vi "LuaVIEW Register and Set Indexed Function.vi"(5 "LuaVIEW reference in":T1, 7 "index":i32, 9 "synopsis":string, 11 "error in (no error)":errorcluster) -> (6 "LuaVIEW reference out":T1, 15 "error out":errorcluster)   [LabVIEW 2012]
doc: "Registers an indexed function with the LuaVIEW state's private function registry and sets the function as part of the state's variable space so that it can be called by name. Indexed functions are functions whose LabVIEW-side functionality is specified via an index instead of a function VI reference. When an indexed function is called, \"LuaVIEW Execute Iteration\" will return and leave the handling to its caller. Thus, indexed functions can be implemented as part of anything that allows selection via an index (typically a case of a case structure)."
uses:
  typedefs/t_LuaVIEW Reference.ctl
  typedefs/et_LuaVIEW CIN Actions.ctl
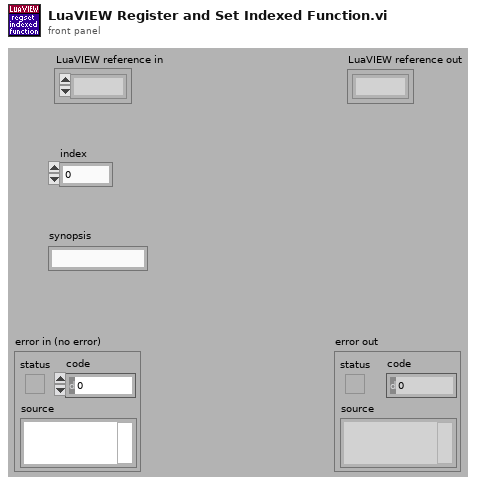
[diagram p1: front panel]
types:
  T1 = typedef "t_LuaVIEW Reference.ctl" = refnum<k1>
  T2 = typedef "et_LuaVIEW CIN Actions.ctl" = enum16{"checksynopsis", "_open", "_registerpublic", "_registerexport", "__never_an_error_result_ns", "luaversion", "cinversion", "_totals", "_taskcount", "pathological", "_unregnextpublic", "registryusecount", "__per_state_actions", "regsetprivate", "regsetindex", "regsetmodule", "_revokeexports", "_usepublic", "prepare", "compile", "execute", "call", "unregstaterefs", "_close", "pullboolean", "pullnumber", "pullI8", "pullU8", "pullI16", "pullU16", "pullI32", "pullU32", "pullobject", "pullrefnum", "pullstring", "pullflat", "pushflat", "pushobject", "getattribute", "setattribute", "stacktostring", "_startyieldtest", "_endyieldtest", "_pollprintbuffer", "__never_an_error_result_ps", "_pollexport", "setclone", "forcecleanup", "gettop", "clearstack", "insert", "pushboolean", "pushnumber", "pushrefnum", "pushstring", "pushnil", "pushvalue", "gettaskref", "settaskref"}
  T3 = typedef "et_LuaVIEW CIN Results.ctl" = enum16{"OK", "error", "main", "call", "clonecall", "modulecall", "exportcall", "index", "yield"}
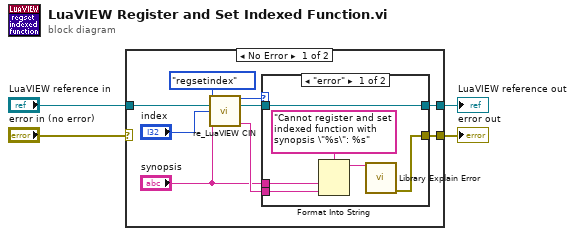
[diagram p0: block diagram]
diagram:
  n1 = case shown="No Error" "error in (no error)" {
    selector: "error in (no error)" -> [_ w22]
    tunnel: [w9 w21] -> w4
    tunnel: [w5 w22] -> w3
    tunnel: "LuaVIEW reference in" -> [w8 w21]
    frame No Error {
      n2 = call "re_LuaVIEW CIN.vi"("action"=et_LuaVIEW_CIN_Actions."regsetindex", "LuaVIEW reference in"=w8, "index in"="index", "string in"="synopsis") -> ("result"=w12:T3, "LuaVIEW reference out"=w10:T1, "string out"=w11:string)  [unwired: 5 in, 4 out]
      n3 = case shown="\"error\"" w12 {
        tunnel: w11 -> [w18 _]
        tunnel: [w19 _] -> w5
        tunnel: "synopsis" -> [w17 _]
        tunnel: w10 -> [w14 w20]
        tunnel: [w14 w20] -> w9
        frame "error" {
          n4 = Format Into String(format string="Cannot register and set indexed function with  synopsis \"%s\": %s", w17, w18) -> (resulting string=w15:string)  [unwired: 2 in, 1 out]
          n5 = call "Library Explain Error.vi"("explanation prefix (none)"=w15) -> ("explained error"=w19:errorcluster)  [unwired: 14 in]
        }
        frame Default {
        }
      }
    }
    frame Error {
    }
  }
  "LuaVIEW reference out" <- w4
  "error out" <- w3
